vi "Write then Read Without Clear.vi"(8 "error in":errorcluster, 10 "write buffer":string, 11 "VISA resource name in":refnum<visa-resource-name>) -> (0 "error out":errorcluster, 1 "Bytes at Port":u32, 2 "read buffer":string, 3 "VISA resource name out":refnum<visa-resource-name>)   [LabVIEW 2018, in "Support Library.lvlib"]
uses:
  Support Library.lvlib
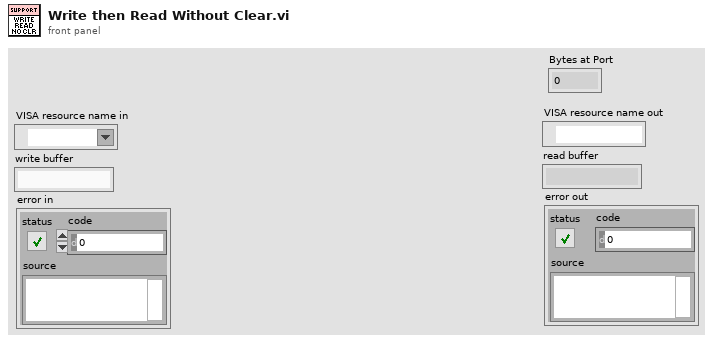
[diagram p1: front panel]
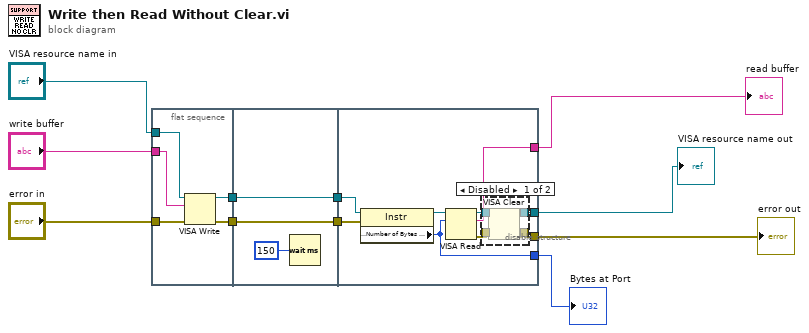
[diagram p0: block diagram]
diagram:
  n1 = flat-sequence {
    tunnel: [w15] -> w11
    tunnel: [w16] -> w10
    tunnel: "write buffer" -> [w14]
    tunnel: "VISA resource name in" -> [w13]
    tunnel: "error in" -> [w12]
    tunnel: w11 -> [w19]
    tunnel: w10 -> [w18]
    tunnel: [w19] -> w9
    tunnel: [w18] -> w8
    tunnel: [w22] -> w7
    tunnel: [w24] -> w5
    tunnel: w9 -> [w23]
    tunnel: w8 -> [w25]
    tunnel: [w21] -> w6
    tunnel: [w20] -> w1
    frame #0 {
      n2 = VISA Write(VISA resource name=w13, write buffer=w14, error in (no error)=w12) -> (VISA resource name out=w16:refnum<visa-resource-name>, error out=w15:errorcluster)  [unwired: 1 out]
    }
    frame #1 {
      n3 = Wait (ms)(milliseconds to wait=u32 150) -> ()  [unwired: 1 out]
    }
    frame #2 {
      n4 = property class="Instr"(reference=w25, error in=w23) -> (reference out=w28:refnum<visa-resource-name>, "Serial Settings:Number of Bytes at Serial Port"=w20:u32)  [unwired: 1 out]
      n5 = VISA Read(VISA resource name=w28, byte count=w20) -> (VISA resource name out=w26:refnum<visa-resource-name>, read buffer=w21:string, error out=w27:errorcluster)  [unwired: 1 in, 1 out]
      n6 = disable-structure shown="Disabled" {
        disable-tunnel: w27 -> [w32 w33]
        disable-tunnel: w26 -> [w31 w34]
        disable-tunnel: [w30 w33] -> w24
        disable-tunnel: [w29 w34] -> w22
        frame Disabled {
          n7 = VISA Clear(VISA resource name=w31, error in (no error)=w32) -> (VISA resource name out=w29:refnum<visa-resource-name>, error out=w30:errorcluster)
        }
        frame Enabled {
        }
      }
    }
  }
  "VISA resource name out" <- w7
  "read buffer" <- w6
  "error out" <- w5
  "Bytes at Port" <- w1
